vi "Element Type.vi"(11 "DoubleControl in":refnum<class "SliderControl.lvclass">) -> (2 "Element Type":string)   [LabVIEW 2020, in "VolatusGUIElements.lvlib" / "SliderControl.lvclass"]
uses:
  SliderControl.lvclass
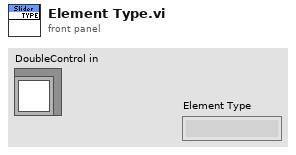
[diagram p1: front panel]
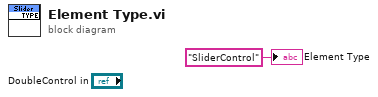
[diagram p0: block diagram]
diagram:
  "Element Type" <- "SliderControl" ("Element Type")
